vi "MEMR-Find Strength.vi"(5 "Metrics":dbl[](array[numeric]), 9 "Level":dbl[](array[numeric])) -> (8 "Strength":dbl)   [LabVIEW 2020]
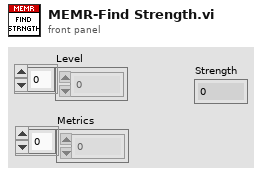
[diagram p1: front panel]
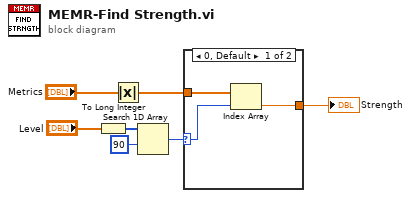
[diagram p0: block diagram]
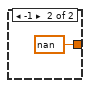
[diagram p2: hidden frame]
diagram:
  n1 = To Long Integer(number="Level") -> (32bit integer=w6:i32[])
  n2 = Absolute Value(x="Metrics") -> (abs(x)=w1:dbl[])
  n3 = Search 1D Array(1D array=w6, element=90) -> (index of element=w4:i32)  [unwired: 1 in]
  n4 = case shown="0, Default" w4 {
    selector: w4 -> [w9 _]
    tunnel: w1 -> [w10 _]
    tunnel: [w8 nan ("dB")] -> w2
    frame 0, Default {
      n5 = Index Array(array=w10, index=w9) -> (element=w8:dbl)
    }
    frame -1 {
    }
  }
  "Strength" <- w2
